vi "FPGAmain_5782_AM_PIDvi.vi"() -> ()   [LabVIEW 2013]
uses:
  FPGA/DataMode.ctl
  FPGA/Input_5782/5782_states.ctl
  <vilib>/Platform/TimedLoop/XDataNode/timing_clust.ctl
  <vilib>/Platform/TimedLoop/XDataNode/nitl_modes.ctl
  <vilib>/Platform/TimedLoop/XDataNode/wakeup.ctl
  <vilib>/rvi/Emulation/niFpgaSctlEmulationGetInTimedLoop.vi
  <vilib>/rvi/Emulation/niFpgaEmulationReportErrorSimple.vi
  <vilib>/rvi/Emulation/niFpgaGetClockAttributes.vi
  <vilib>/rvi/eio/common/nirviEmuTemplateMethod_errors.vi
  <vilib>/rvi/Emulation/niFpgaCriticalErrorInLSC.vi
  <vilib>/rvi/DataTransferAndStorage/Register/Emulation/niFpgaRegisterEmulationFpgaImpl.vi
  <instcachedir>/0/niFpgaRegisterEmulationFpgaImpl_DCF4BC0110594B98B44A971D60CEEC4D.lvgen/niFpgaRegisterEmulationFpgaImpl_DCF4BC0110594B98B44A971D60CEEC4D_003.vi
  <vilib>/rvi/DataTransferAndStorage/Container/Common/niFpgaContainerGetUniqueNameForEmu.vi
  <instcachedir>/0/niFpgaRegisterEmulationFpgaImpl_DCF4BC0110594B98B44A971D60CEEC4D.lvgen/niFpgaRegisterEmulationFpgaImpl_DCF4BC0110594B98B44A971D60CEEC4D_021.vi
  <instcachedir>/0/niFpgaRegisterEmulationFpgaImpl_DCF4BC0110594B98B44A971D60CEEC4D.lvgen/niFpgaRegisterEmulationFpgaImpl_DCF4BC0110594B98B44A971D60CEEC4D_020.vi
  <instcachedir>/0/niFpgaRegisterEmulationFpgaImpl_DCF4BC0110594B98B44A971D60CEEC4D.lvgen/niFpgaRegisterEmulationFpgaImpl_DCF4BC0110594B98B44A971D60CEEC4D_016.vi
  <instcachedir>/0/niFpgaRegisterEmulationFpgaImpl_DCF4BC0110594B98B44A971D60CEEC4D.lvgen/niFpgaRegisterEmulationFpgaImpl_DCF4BC0110594B98B44A971D60CEEC4D_010.vi
  <instcachedir>/0/niFpgaRegisterEmulationFpgaImpl_DCF4BC0110594B98B44A971D60CEEC4D.lvgen/niFpgaRegisterEmulationFpgaImpl_DCF4BC0110594B98B44A971D60CEEC4D_009.vi
  <vilib>/rvi/FIFO/Fifo_Resource/nirvififoEmulationReadFpgaImpl.vi
  <vilib>/rvi/interface/RandomDataEmulation/nirviRandomDataMultiElementFPGAFIFO.vi
  <instcachedir>/0/nirviRandomDataMultiElementFPGAFIFO_F2B80EDE0D7944A08478D8D26097D4DB.lvgen/nirviRandomDataMultiElementFPGAFIFO_F2B80EDE0D7944A08478D8D26097D4DB_005.vi
  <vilib>/rvi/interface/RandomDataEmulation/niFpgaRandomDataHandleErrors.vi
  <instcachedir>/0/niFpgaRegisterEmulationFpgaImpl_DCF4BC0110594B98B44A971D60CEEC4D.lvgen/niFpgaRegisterEmulationFpgaImpl_DCF4BC0110594B98B44A971D60CEEC4D_013.vi
  <vilib>/rvi/interface/RandomDataEmulation/nirviRandomDataFPGAFIFO.vi
  <vilib>/rvi/FIFO/Fifo_Resource/nirvififoEmulationWriteFpgaImpl.vi
  <vilib>/Platform/TimedLoop/XDataNode/XDataNode.xnode
  <vilib>/eio/EIONode/EIONode.xnode
  <vilib>/rvi/DataTransferAndStorage/Container/XNode/niFpgaContainer.xnode
  <vilib>/rvi/DataTransferAndStorage/Register/Emulation/niFpgaRegisterEmulation.vi
  <vilib>/rvi/FIFO/Fifo_Resource/nirvififoEmulationRead.vi
  <vilib>/rvi/interface/RandomDataEmulation/nirviRandomDataFpgaMultiElementTemplate.vi
  <vilib>/rvi/interface/RandomDataEmulation/nirviRandomDataFpgaReadWriteTemplate.vi
  <vilib>/rvi/FIFO/Fifo_Resource/nirvififoEmulationWrite.vi
  <vilib>/Platform/TimedLoop/XDataNode/XDNodeRunTimeDep.lvlib
panel:
  in  "AM phase":fxp<+,64,64>
  in  "delay phase":fxp<+,64,64>
  in  "User Command Commit":bool
  in  "User Command":u8
  out "User Command Idle":bool
  out "User Command Status":u8
  in  "User Data 0":u8
  in  "User Data 1":u8
  out "PLL Locked":bool
  out "User Error":bool
  out "Configured?":bool
  in  "Continuous":bool
  in  "5782 record length":u16=4000 caption="Samples Per Trigger" min=1 step=1
  in  "Trigger Acquisition":bool
  out "IO Module\\Trigger Input":bool
  in  "Downsample":fxp<+,8,8>=1.0
  in  "new coeffs":bool
  in  "FIR coeffs":fxp<+/-,18,18>[](array[numeric])
  in  "CIC Gain":fxp<+/-,32,1>=0.00390625 format="%#_32g"
  in  "Acquisition running":bool
  in  "Phase output":fxp<+,64,64>[](array[numeric])=[0.0, 0.0, 0.0, 0.0, 0.0, 0.0, 0.0, 0.0]
  in  "Simulated phase 5782":fxp<+,64,64>[](array[numeric])=[0.0, 0.0]
  in  "Mode":T1
  in  "Phase 5782":fxp<+,64,64>[](array[numeric])=[0.0, 0.0]
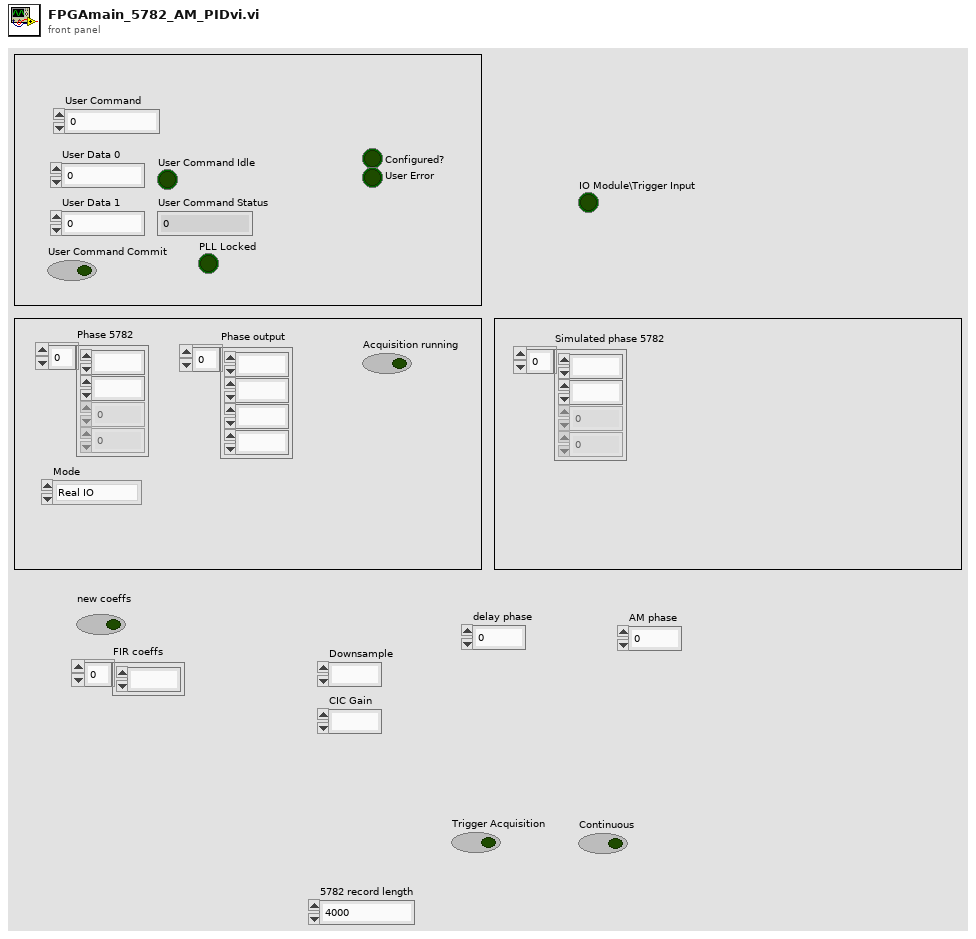
[diagram p1: front panel]
types:
  T1 = typedef "DataMode.ctl" = enum16{"Real IO", "Simulated"}
  T2 = typedef "5782_states.ctl" = enum8{"Wait for trigger", "Acquisition", "Send record length", "Quiet period"}
  T3 = typedef "XDNodeRunTimeDep.lvlib/timing_clust.ctl" = cluster{"Expected End [f-1]":u64, "Actual End [f-1]":u64, "Finished Late? [f-1]":bool, "Expected End [i-1]":u64, "Actual End [i-1]":u64, "Finished Late? [i-1]":bool, "Expected Start [i]":u64, "Actual Start [i]":u64, "Expected Start [f]":u64, "Actual Start [f]":u64, "Source Name":string, "Structure Name":string, "Period":i64, "Deadline":i64, "Offset":i64, "Start":i64, "Priority":i32, "Timeout":i32, "Mode":T4, "Wakeup Reason":T5, "Error":errorcluster, "Source Type":string, "Secondary Source Type":string, "Global End Time":u64, "Global Start Time":u64, "Frame Duration":u64, "Iteration Duration":u64, "Assigned CPU":i32, "I/O Scan Engine Mode":u32}
  T4 = typedef "XDNodeRunTimeDep.lvlib/nitl_modes.ctl" = enum32{"No Change", "Process missed periods, maintain original phase", "Discard missed periods, maintain original phase", "Process missed periods, ignore original phase", "Discard missed periods, ignore original phase"}
  T5 = typedef "XDNodeRunTimeDep.lvlib/wakeup.ctl" = enum32{"Normal", "Aborted", "Asynchronous wakeup", "Timing source error", "Timed loop error", "Timeout"}
  T6 = typedef "I16 array size 2.ctl" = i16[]
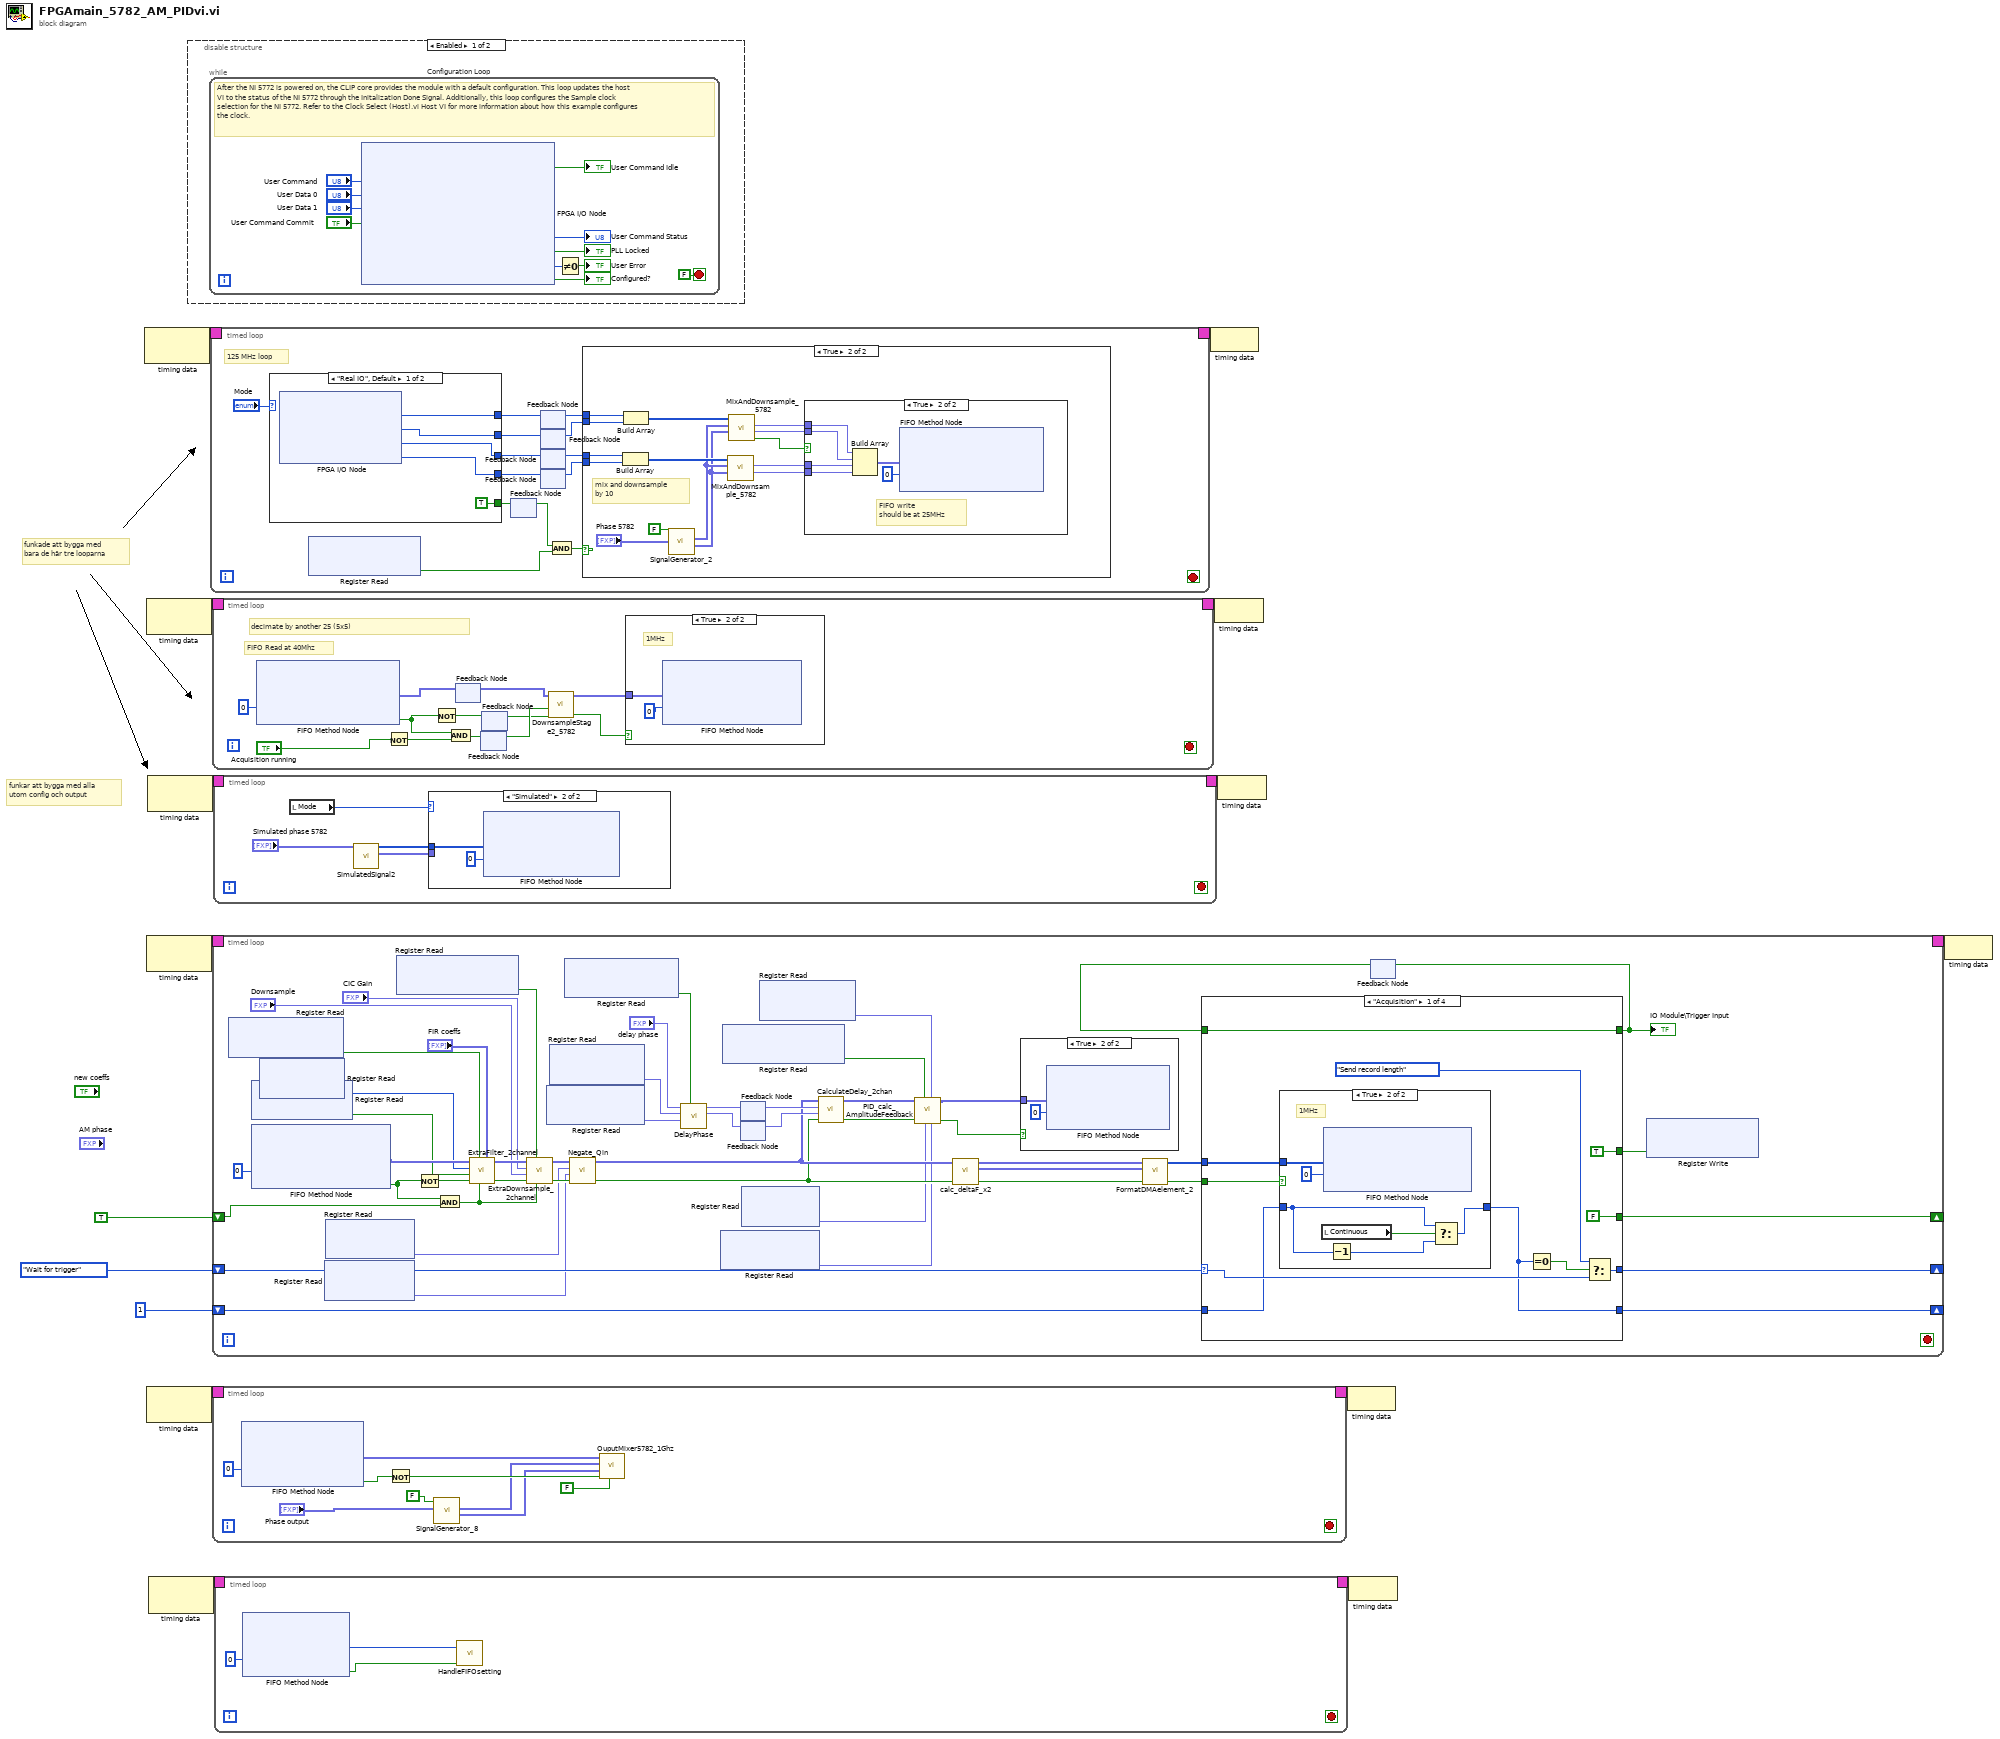
[diagram p0: block diagram]
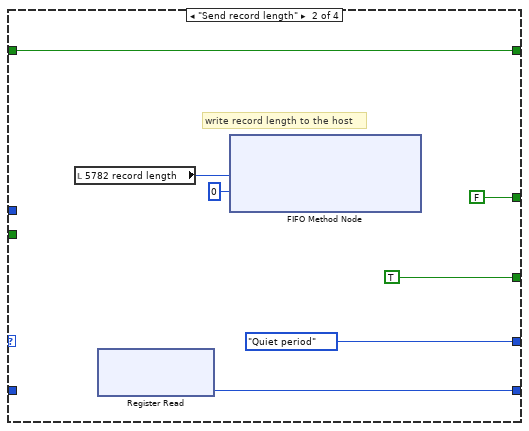
[diagram p4: hidden frame]
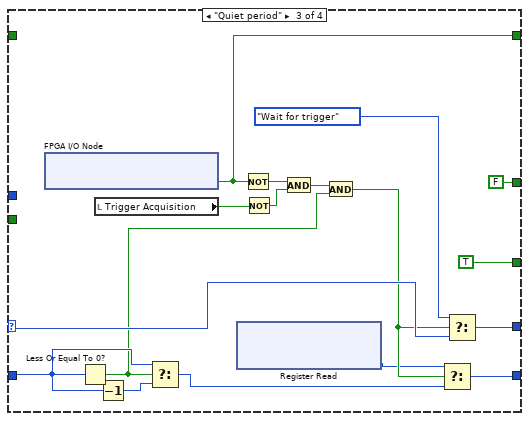
[diagram p5: hidden frame]
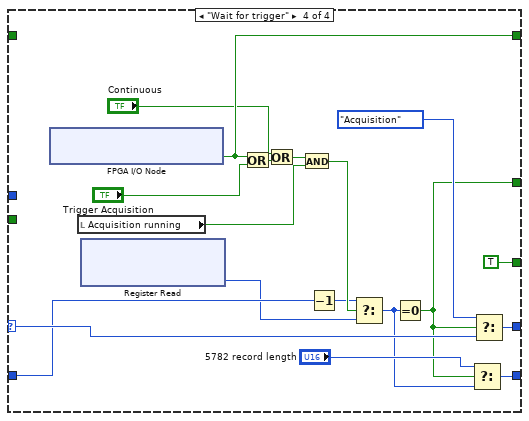
[diagram p6: hidden frame]
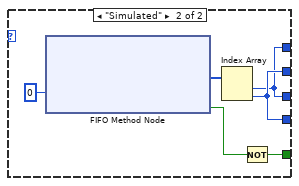
[diagram p10: hidden frame]
diagram:
  # "funkar att bygga med alla\nutom config och output"
  # "funkade att bygga med\nbara de här tre looparna"
  n1 = node-c288() -> (w11:T3)  [unwired: 1 in]
  n2 = node-c288() -> (w15:T3)  [unwired: 1 in]
  n3 = node-c288() -> (w9:T3)  [unwired: 1 in]
  n4 = node-c288() -> (w2:T3)  [unwired: 1 in]
  n5 = node-c288() -> (w13:T3)  [unwired: 1 in]
  n6 = node-c288() -> (w4:T3)  [unwired: 1 in]
  n7 = disable-structure shown="Enabled" {
    frame Enabled {
      n8 = while "Configuration Loop" {
        stop <- FALSE stop-if-true
        # "After the NI 5772 is powered on, the CLIP core provides the module with a default configuration. This loop updates the host VI to the status of the NI 5772 through the Initalization Done Signal. Additionally, this loop configures the Sample clock selection for the NI 5772. Refer to the Clock Select (Host).vi Host VI for more information about how this example configures the clock."
        n9 = xnode "FPGA I/O Node"("IO Module\\User Command"="User Command", "IO Module\\User Data 0"="User Data 0", "IO Module\\User Data 1"="User Data 1", "IO Module\\User Command Commit"="User Command Commit") -> ("IO Module\\User Command Idle"=→"User Command Idle":bool, "IO Module\\User Command Status"=→"User Command Status":u8, "IO Module\\PLL Locked"=→"PLL Locked":bool, "IO Module\\User Error"=w21:u8, "IO Module\\Initialization Done"=→"Configured?":bool)  [unwired: 9 in, 9 out]
        n10 = Not Equal To 0?(x=w21) -> (x != 0?=→"User Error":bool)
      }
    }
    frame Disabled {
    }
  }
  n11 = timed-loop {
    timing: w11 -> [_]
    timing-out: [_] -> w10
    stop <- _ stop-if-true
    # "125 MHz loop"
    n12 = case shown="\"Real IO\", Default" "Mode" {
      tunnel: [w65 w68] -> w37
      tunnel: [w64 w69] -> w35
      tunnel: [w63 w68] -> w33
      tunnel: [w62 w69] -> w30
      tunnel: [TRUE w66] -> w29
      frame "Real IO", Default {
        n13 = xnode "FPGA I/O Node"() -> ("IO Module\\AI 0 N-1"=w65:i16, "IO Module\\AI 0 N"=w64:i16, "IO Module\\AI 1 N-1"=w63:i16, "IO Module\\AI 1 N"=w62:i16)  [unwired: 4 in, 4 out]
      }
      frame "Simulated" {
        n14 = xnode ("FIFO Method Node")("Timeout"=0) -> ("Element"=w70:i16[], "Timed Out?"=w67:bool)  [unwired: 1 in, 1 out]
        n15 = Index Array(array=w70) -> (element #1=w68:i16, element #2=w69:i16)  [unwired: 2 in]
        n16 = Not(x=w67) -> (.not. x?=w66:bool)
      }
    }
    n17 = xnode ("Register Read")() -> ("Data"=w27:bool)  [unwired: 1 in, 1 out]
    n18 = feedback #1() -> (w28:bool)  [unwired: 1 in]
    n19 = feedback-in #1(w29) -> ()
    n20 = feedback #2() -> (w36:i16)  [unwired: 1 in]
    n21 = feedback-in #2(w37) -> ()
    n22 = feedback #3() -> (w34:i16)  [unwired: 1 in]
    n23 = feedback-in #3(w35) -> ()
    n24 = feedback #4() -> (w32:i16)  [unwired: 1 in]
    n25 = feedback-in #4(w33) -> ()
    n26 = feedback #5() -> (w31:i16)  [unwired: 1 in]
    n27 = feedback-in #5(w30) -> ()
    n28 = And(x=w28, y=w27) -> (x .and. y?=w38:bool)
    n29 = case shown="True" w38 {
      tunnel: w36 -> [_ w45]
      tunnel: w34 -> [_ w44]
      tunnel: w32 -> [_ w43]
      tunnel: w31 -> [_ w42]
      frame False {
      }
      frame True {
        # "mix and downsample\nby 10"
        n30 = Build Array(w43, w42) -> (w54:i16[])
        n31 = Build Array(w45, w44) -> (w41:i16[])
        n32 = call "SignalGenerator_2.vi"("Phase"="Phase 5782", "reset"=FALSE) -> ("Sine out"=w46:fxp<+/-,16,0>[], "Cosine out"=w47:fxp<+/-,16,0>[])  [unwired: 8 in]
        n33 = call "MixAndDownsample_5782.vi"("Sine in"=w46, "Cosine in"=w47, "Signal Input"=w54) -> ("Q out"=w49:fxp<+/-,16,14>, "I out"=w50:fxp<+/-,16,14>)  [unwired: 6 in, 1 out]
        n34 = call "MixAndDownsample_5782.vi"("Sine in"=w46, "Cosine in"=w47, "Signal Input"=w41) -> ("data valid"=w51:bool, "Q out"=w52:fxp<+/-,16,14>, "I out"=w53:fxp<+/-,16,14>)  [unwired: 6 in]
        n35 = case shown="True" w51 {
          tunnel: w52 -> [_ w60]
          tunnel: w53 -> [_ w57]
          tunnel: w50 -> [_ w56]
          tunnel: w49 -> [_ w55]
          frame False {
          }
          frame True {
            # "FIFO write\nshould be at 25MHz"
            n36 = Build Array(w57, w60, w56, w55) -> (w59:fxp<+/-,16,14>[])
            n37 = xnode ("FIFO Method Node")("Element"=w59, "Timeout"=0) -> ()  [unwired: 1 in, 2 out]
          }
        }
      }
    }
  }
  n38 = timed-loop {
    timing: w15 -> [_]
    timing-out: [_] -> w14
    stop <- _ stop-if-true
    # "FIFO Read at 40Mhz"
    # "decimate by another 25 (5x5)"
    n39 = xnode ("FIFO Method Node")("Timeout"=0) -> ("Element"=w79:fxp<+/-,16,14>[], "Timed Out?"=w81:bool)  [unwired: 1 in, 1 out]
    n40 = Not(x="Acquisition running") -> (.not. x?=w82:bool)
    n41 = Not(x=w81) -> (.not. x?=w75:bool)
    n42 = And(x=w81, y=w82) -> (x .and. y?=w77:bool)
    n43 = feedback #6() -> (w78:fxp<+/-,16,14>[])  [unwired: 1 in]
    n44 = feedback-in #6(w79) -> ()
    n45 = feedback #7() -> (w76:bool)  [unwired: 1 in]
    n46 = feedback-in #7(w77) -> ()
    n47 = feedback #8() -> (w74:bool)  [unwired: 1 in]
    n48 = feedback-in #8(w75) -> ()
    n49 = call "DownsampleStage2_5782.vi"("valid in"=w74, "reset"=w76, "Data in"=w78) -> ("valid out"=w83:bool, "data out"=w84:fxp<+/-,16,14>[])  [unwired: 7 in]
    n50 = case shown="True" w83 {
      tunnel: w84 -> [_ w86]
      frame False {
      }
      frame True {
        # "1MHz"
        n51 = xnode ("FIFO Method Node")("Element"=w86, "Timeout"=0) -> ()  [unwired: 1 in, 2 out]
      }
    }
  }
  n52 = timed-loop {
    timing: w9 -> [_]
    timing-out: [_] -> w8
    shift-right: [w137] -> _
    shift-left: 5782_states."Wait for trigger" ("5782 states") -> [w139]
    shift-right: [w136] -> _
    shift-left: u16 1 ("trigger samples") -> [w138]
    shift-right: [w122] -> _
    shift-left: TRUE -> [w125]
    stop <- _ stop-if-true
    n53 = xnode ("Register Read")() -> ("Data"=w106:bool)  [unwired: 1 in, 1 out]
    n54 = xnode ("Register Read")() -> ("Data"=w98:bool)  [unwired: 1 in, 1 out]
    n55 = xnode ("FIFO Method Node")("Timeout"=0) -> ("Element"=w127:fxp<+/-,16,14>[], "Timed Out?"=w126:bool)  [unwired: 1 in, 1 out]
    n56 = xnode ("Register Read")() -> ("Data"=w99:i32)  [unwired: 1 in, 1 out]
    n57 = xnode ("Register Read")() -> ("Data"=w104:fxp<+/-,16,14>)  [unwired: 1 in, 1 out]
    n58 = xnode ("Register Read")() -> ("Data"=w105:fxp<+/-,16,14>)  [unwired: 1 in, 1 out]
    n59 = xnode ("Register Read")() -> ("Data"=w100:bool)  [unwired: 1 in, 1 out]
    n60 = Not(x=w126) -> (.not. x?=w132:bool)
    n61 = And(x=w126, y=w125) -> (x .and. y?=w134:bool)
    n62 = call "ExtraFilter_2channel.vi"(5:"new coeffs"="FIR coeffs", "reset"=w134, 7:"new coeffs"=w106, "valid in"=w132, "enable filter"=w98, "new shift"=w99, "Data in"=w127) -> ("valid out"=w133:bool, "Data out"=w131:fxp<+/-,16,14>[])  [unwired: 3 in]
    n63 = call "ExtraDownsample_2channel.vi"("reset"=w134, "Set downsample"=w100, "valid in"=w133, "Downsample"="Downsample", "CIC Gain"="CIC Gain", "Data in"=w131) -> ("valid out"=w117:bool, "Data out"=w118:fxp<+/-,16,14>[])  [unwired: 4 in]
    n64 = xnode ("Register Read")() -> ("Data"=w101:fxp<+/-,16,0>)  [unwired: 1 in, 1 out]
    n65 = xnode ("Register Read")() -> ("Data"=w102:fxp<+/-,16,0>)  [unwired: 1 in, 1 out]
    n66 = xnode ("Register Read")() -> ("Data"=w103:bool)  [unwired: 1 in, 1 out]
    n67 = call "Negate_Qin.vi"("valid in"=w117, "DC offset chan 1"=w104, "DC offset chan 0"=w105, "Data in"=w118) -> ("valid out"=w109:bool, "Data out"=w114:fxp<+/-,16,14>[])  [unwired: 6 in]
    n68 = call "DelayPhase.vi"("Use fixed delay"=w103, "fixed cos_fi"=w101, "fixed sin fi"=w102, "delay phase"="delay phase") -> ("cos_fi"=w111:fxp<+/-,16,0>, "sin fi"=w112:fxp<+/-,16,0>)  [unwired: 6 in]
    n69 = xnode "Register Read"() -> ("Data"=w91:fxp<+/-,32,6>)  [unwired: 1 in, 1 out]
    n70 = xnode "Register Read"() -> ("Data"=w93:bool)  [unwired: 1 in, 1 out]
    n71 = feedback-in #9(w112) -> ()
    n72 = feedback #9() -> (w116:fxp<+/-,16,0>)  [unwired: 1 in]
    n73 = feedback #10() -> (w115:fxp<+/-,16,0>)  [unwired: 1 in]
    n74 = feedback-in #10(w111) -> ()
    n75 = xnode "Register Read"() -> ("Data"=w92:fxp<+/-,32,6>)  [unwired: 1 in, 1 out]
    n76 = xnode "Register Read"() -> ("Data"=w90:fxp<+/-,32,6>)  [unwired: 1 in, 1 out]
    n77 = call "CalculateDelay_2chan.vi"("input valid"=w109, "cos_fi"=w115, "sin fi"=w116, "Data in"=w114) -> ("output valid"=w95:bool, "Data out"=w96:fxp<+/-,16,14>[])  [unwired: 6 in]
    n78 = call "PID_calc_AmplitudeFeedback.vi"("Kd/Tau"=w91, "Ki*Tau"=w90, "Kp"=w92, "Enabled"=w93, "input valid"=w95, "Data in"=w96) -> ("output valid"=w94:bool, "data out"=w97:fxp<+/-,16,14>[])  [unwired: 2 in, 2 out]
    n79 = call "calc_deltaF_x2.vi"("valid in"=w109, "Data in"=w114) -> ("valid out"=w108:bool, "deltaF"=w107:fxp<+/-,32,30>[], "Data out"=w110:fxp<+/-,16,14>[])  [unwired: 7 in]
    n80 = case shown="True" w94 {
      tunnel: w97 -> [_ w140]
      frame False {
      }
      frame True {
        n81 = xnode ("FIFO Method Node")("Element"=w140, "Timeout"=0) -> ()  [unwired: 1 in, 2 out]
      }
    }
    n82 = call "FormatDMAelement_2.vi"("valid in"=w108, "deltaF"=w107, "Data in"=w110) -> ("valid out"=w123:bool, "Element"=w124:u64[])  [unwired: 7 in]
    n83 = feedback #11() -> (w120:bool)  [unwired: 1 in]
    n84 = case shown="\"Acquisition\"" w139 {
      selector: w139 -> [w152 _ w182 w201]
      tunnel: w138 -> [w148 _ w170 w188]
      tunnel: [w151 5782_states."Quiet period" ("5782 states") w181 w200] -> w137
      tunnel: [w145 w160 w183 w199] -> w136
      tunnel: w124 -> [w146 _ _ _]
      tunnel: w123 -> [w147 _ _ _]
      tunnel: [FALSE TRUE TRUE TRUE] -> w122
      tunnel: [TRUE FALSE ("5782 triggered") FALSE ("5782 triggered") w192] -> w121
      tunnel: [w144 w161 w172 w191] -> w119
      tunnel: w120 -> [w144 w161 _ _]
      frame "Acquisition" {
        n85 = case shown="True" w147 {
          tunnel: w146 -> [_ w159]
          tunnel: [w153 w156] -> w145
          tunnel: w148 -> [w153 w154]
          frame False {
          }
          frame True {
            # "1MHz"
            n86 = local read "Continuous"() -> (w157:bool)
            n87 = xnode ("FIFO Method Node")("Element"=w159, "Timeout"=0) -> ()  [unwired: 1 in, 2 out]
            n88 = Decrement(x=w154) -> (x-1=w155:u16)
            n89 = Select(t=w154, s=w157, f=w155) -> (s? t:f=w156:u16)
          }
        }
        n90 = Equal To 0?(x=w145) -> (x = 0?=w149:bool)
        n91 = Select(t=5782_states."Send record length" ("5782 states"), s=w149, f=w152) -> (s? t:f=w151:T2)
      }
      frame "Send record length" {
        # "write record length to the host"
        n92 = local read "5782 record length"() -> (w163:u16)
        n93 = xnode ("Register Read")() -> ("Data"=w160:u16)  [unwired: 1 in, 1 out]
        n94 = xnode ("FIFO Method Node")("Element"=w163, "Timeout"=0) -> ()  [unwired: 1 in, 2 out]
      }
      frame "Quiet period" {
        n95 = xnode "FPGA I/O Node"() -> ("IO Module\\Trigger Input"=w172:bool)  [unwired: 1 in, 1 out]
        n96 = Less Or Equal To 0?(x=w170) -> (x <= 0?=w169:bool)
        n97 = local read "Trigger Acquisition"() -> (w178:bool)
        n98 = Decrement(x=w170) -> (x-1=w171:u16)
        n99 = Select(t=w170, s=w169, f=w171) -> (s? t:f=w168:u16)
        n100 = xnode ("Register Read")() -> ("Data"=w167:u16)  [unwired: 1 in, 1 out]
        n101 = Not(x=w172) -> (.not. x?=w177:bool)
        n102 = Not(x=w178) -> (.not. x?=w176:bool)
        n103 = And(x=w177, y=w176) -> (x .and. y?=w175:bool)
        n104 = And(x=w175, y=w169) -> (x .and. y?=w180:bool)
        n105 = Select(t=w167, s=w180, f=w168) -> (s? t:f=w183:u16)
        n106 = Select(t=5782_states."Wait for trigger" ("5782 states"), s=w180, f=w182) -> (s? t:f=w181:T2)
      }
      frame "Wait for trigger" {
        n107 = xnode "FPGA I/O Node"() -> ("IO Module\\Trigger Input"=w191:bool)  [unwired: 1 in, 1 out]
        n108 = local read "Acquisition running"() -> (w193:bool)
        n109 = xnode ("Register Read")() -> ("Data"=w184:u16)  [unwired: 1 in, 1 out]
        n110 = Or(x=w191, y="Trigger Acquisition") -> (x .or. y?=w187:bool)
        n111 = Or(x="Continuous", y=w187) -> (x .or. y?=w185:bool)
        n112 = And(x=w185, y=w193) -> (x .and. y?=w194:bool)
        n113 = Decrement(x=w188) -> (x-1=w189:u16)
        n114 = Select(t=w189, s=w194, f=w184) -> (s? t:f=w190:u16)
        n115 = Equal To 0?(x=w190) -> (x = 0?=w192:bool)
        n116 = Select(t="5782 record length", s=w192, f=w190) -> (s? t:f=w199:u16)
        n117 = Select(t=5782_states."Acquisition" ("5782 states"), s=w192, f=w201) -> (s? t:f=w200:T2)
      }
    }
    "IO Module\\Trigger Input" <- w119
    n118 = feedback-in #11(w119) -> ()
    n119 = xnode ("Register Write")("Data"=w121) -> ()  [unwired: 1 in, 1 out]
  }
  n120 = timed-loop {
    timing: w2 -> [_]
    timing-out: [_] -> w1
    stop <- _ stop-if-true
    n121 = xnode ("FIFO Method Node")("Timeout"=0) -> ("Element"=w208:fxp<+/-,16,14>[], "Timed Out?"=w211:bool)  [unwired: 1 in, 1 out]
    n122 = Not(x=w211) -> (.not. x?=w207:bool)
    n123 = call "SignalGenerator_8.vi"("Phase"="Phase output", "reset"=FALSE) -> ("Sine out"=w204:fxp<+/-,16,0>[], "Cosine out"=w205:fxp<+/-,16,0>[])  [unwired: 8 in]
    n124 = call "OuputMixer5782_1Ghz.vi"("reset"=FALSE, "valid in"=w207, "Sine in"=w204, "Cosine in"=w205, "Data in"=w208) -> ()  [unwired: 5 in, 2 out]
  }
  n125 = timed-loop {
    timing: w13 -> [_]
    timing-out: [_] -> w12
    stop <- _ stop-if-true
    n126 = local read "Mode"() -> (w218:T1)
    n127 = call "SimulatedSignal2.vi"("Phase"="Simulated phase 5782") -> ("dummy do not use"=w215:fxp<+/-,16,0>[], "output"=w217:T6)  [unwired: 9 in]
    n128 = case shown="\"Simulated\"" w218 {
      tunnel: w217 -> [_ w219]
      tunnel: w215 -> [_ _]
      frame "Real IO", Default {
      }
      frame "Simulated" {
        n129 = xnode ("FIFO Method Node")("Element"=w219, "Timeout"=0) -> ()  [unwired: 1 in, 2 out]
      }
    }
  }
  n130 = timed-loop {
    timing: w4 -> [_]
    timing-out: [_] -> w3
    stop <- _ stop-if-true
    n131 = xnode ("FIFO Method Node")("Timeout"=0) -> ("Element"=w224:u64, "Timed Out?"=w223:bool)  [unwired: 1 in, 1 out]
    n132 = call "HandleFIFOsetting.vi"("timed out"=w223, "Value"=w224) -> ()  [unwired: 10 in]
  }
  n133 = node-c288(w10) -> ()
  n134 = node-c288(w14) -> ()
  n135 = node-c288(w12) -> ()
  n136 = node-c288(w1) -> ()
  n137 = node-c288(w3) -> ()
  n138 = node-c288(w8) -> ()
